vi "_Main_01.vi"() -> ()   [LabVIEW 2017]
uses:
  <vilib>/Instr/_visa.llb/VISA Configure Serial Port (Instr).vi
  <vilib>/Analysis/NI_AALBase.lvlib
panel:
  in  "Numeric":dbl min=0.0 max=11.73
  in  "OK Button":bool
  out "3 sd":dbl format="%0.2f"
  out "mean":dbl format="%0.2f"
  out "TrigTimer, s":dbl
  out "Histogram Graph":T1(graph)
  out "temp":dbl format="%#.2g"
  out "serv1":i32
  out "serv2":i32
  out "serv3":i32
  out "serv4":i32
  out "Vout, V":dbl format="%#.2g"
  out "Vin, V":dbl format="%#.3g"
  out "Temp, K":dbl
  out "Temp_sp, K":dbl
  out "Temp_gsp, K":dbl
  out "Field LOG":cluster{dbl[], dbl[]}(graph)
  out "Bytes at Port":u32
  out "RecTry":i32
  in  "Stop Button":bool
  in  "COM port":refnum<visa-resource-name>
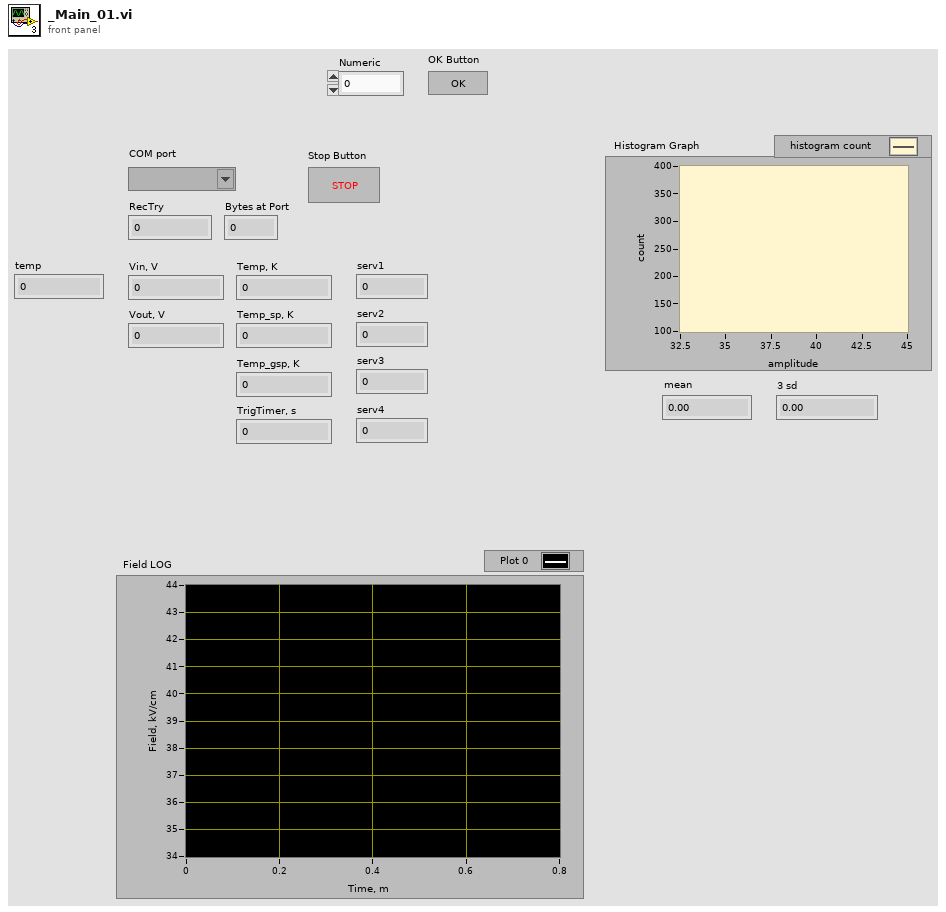
[diagram p1: front panel]
types:
  T1 = cluster{"X Values":dbl[], "Histogram: h(x)":i32[]}
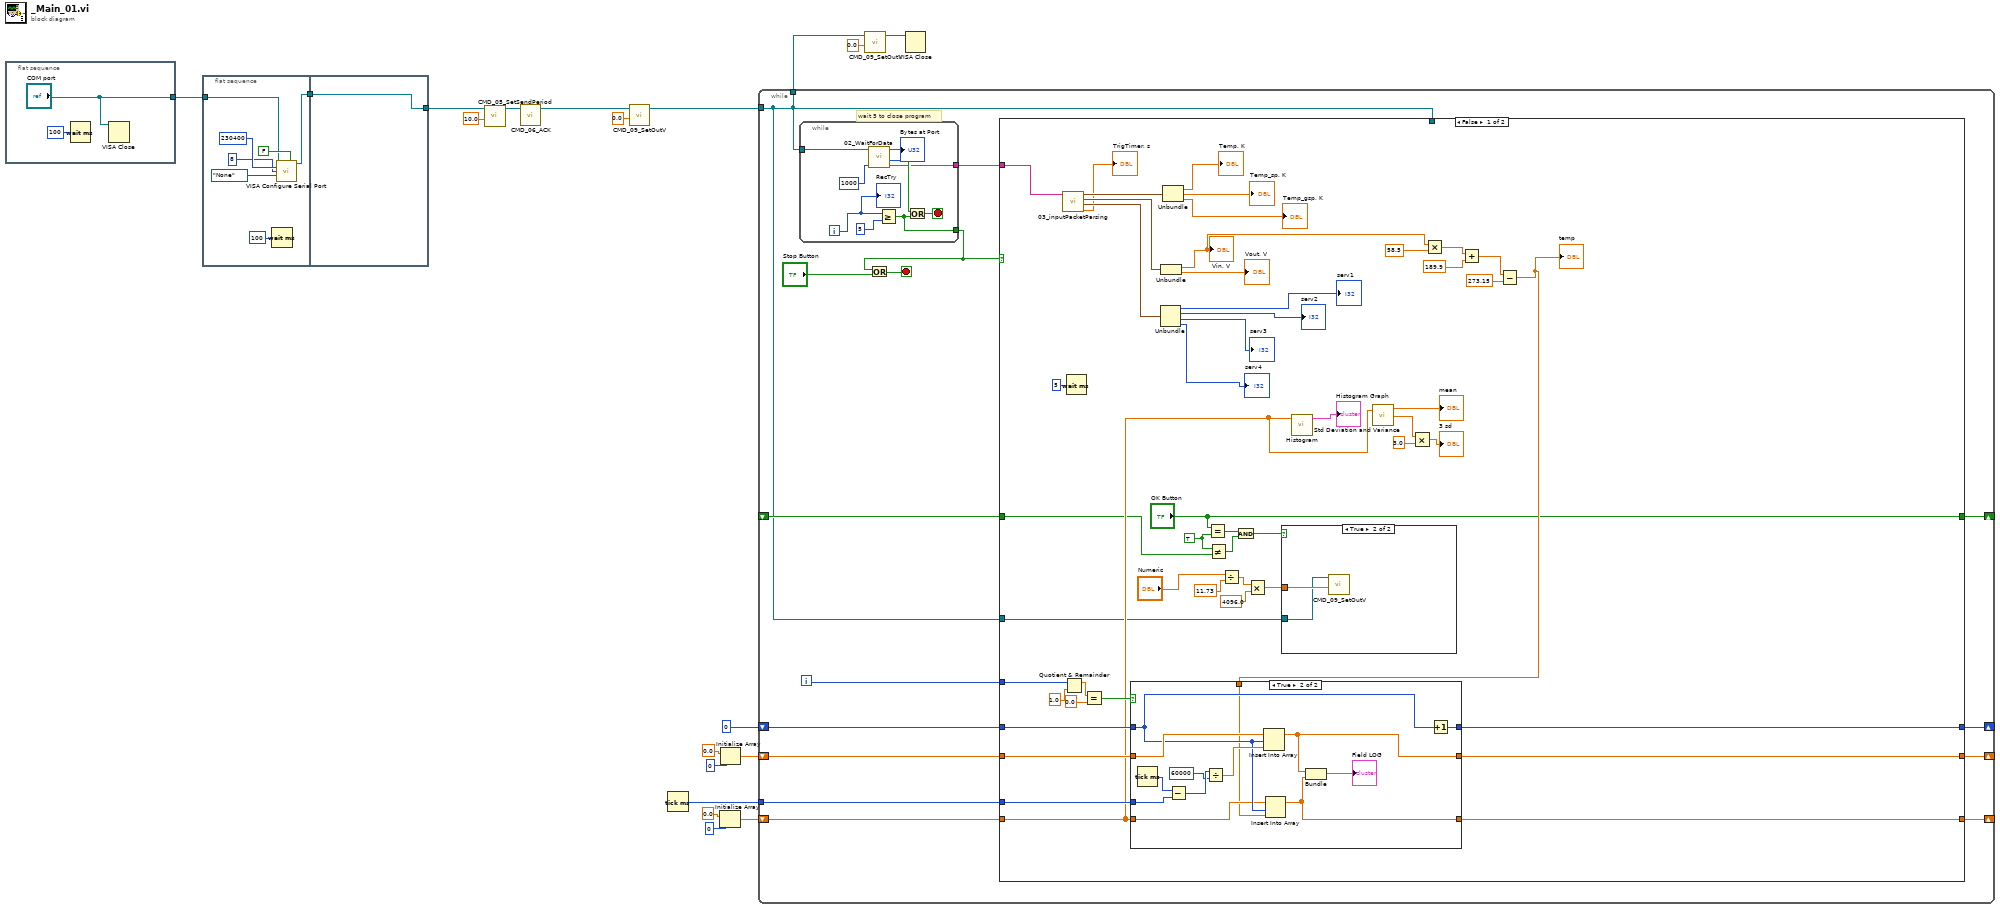
[diagram p0: block diagram]
diagram:
  n1 = flat-sequence {
    tunnel: ["COM port"] -> w19
    frame #0 {
      n2 = Wait (ms)(milliseconds to wait=u32 100) -> ()  [unwired: 1 out]
      n3 = VISA Close(VISA resource name="COM port") -> ()  [unwired: 1 in, 1 out]
    }
  }
  n4 = flat-sequence {
    tunnel: w19 -> [w24]
    tunnel: [w23] -> w16
    tunnel: [w29] -> w7
    tunnel: w16 -> [w29]
    frame #0 {
      n5 = Wait (ms)(milliseconds to wait=u32 100) -> ()  [unwired: 1 out]
      n6 = call-poly "VISA Configure Serial Port"("VISA resource name"=w24, "Enable Termination\nChar (T)"=FALSE ("Enable Termination\nChar (T)"), "baud rate (9600)"=u32 230400, "data bits (8)"=u16 8, "parity (0:none)"=enum16{"None", "Odd", "Even", "Mark", "Space"}."None") -> ("VISA resource name out"=w23:refnum<visa-resource-name>)  [unwired: 9 in, 1 out]
    }
    frame #1 {
    }
  }
  n7 = call "CMD_05_SetSendPeriod.vi"("Period, ms"=10.0, "VISA resource name"=w7) -> ("VISA resource name out"=w17:refnum<visa-resource-name>)  [unwired: 9 in]
  n8 = call "CMD_06_ACK.vi"("VISA resource name"=w17) -> ("VISA resource name out"=w1:refnum<visa-resource-name>)  [unwired: 10 in]
  n9 = call "CMD_09_SetOutV.vi"("Voltage, d"=0.0, "VISA resource name"=w1) -> ("VISA resource name out"=w2:refnum<visa-resource-name>)  [unwired: 9 in]
  n10 = Tick Count (ms)() -> (millisecond timer value=w11:u32)
  n11 = Initialize Array(0.0 ("element"), 0 ("dimension size")) -> (w8:dbl[])
  n12 = Initialize Array(0.0 ("element"), 0 ("dimension size")) -> (w12:dbl[])
  n13 = while {
    tunnel: w2 -> [w30]
    tunnel: [w30] -> w5
    shift-right: [w39] -> _
    shift-left: 0 -> [w40]
    tunnel: w11 -> [w37]
    shift-right: [w35] -> _
    shift-left: w12 -> [w38]
    shift-right: [w34] -> _
    shift-left: w8 -> [w36]
    shift-right: [w32] -> _
    shift-left: _ -> [w31]
    i -> [w41]
    stop <- w44 stop-if-true
    # "wait 5 to close program"
    n14 = while {
      tunnel: w30 -> [w117]
      tunnel: [w120] -> w43
      tunnel: [w121] -> w42
      i -> [w119]
      stop <- w123 stop-if-true
      n15 = call "02_WaitForData.vi"("WaitTimeoutMS"=u32 1000, "VISA"=w117) -> ("Buffer"=w121:string, "Bytes at Port"=→"Bytes at Port":u32, "Data Recived"=w122:bool)  [unwired: 7 in]
      n16 = Greater Or Equal?(x=w119, y=5) -> (x >= y?=w120:bool)
      n17 = Or(x=w122, y=w120) -> (x .or. y?=w123:bool)
      "RecTry" <- w119
    }
    n18 = Or(x=w43, y="Stop Button") -> (x .or. y?=w44:bool)
    n19 = case shown="False" w43 {
      tunnel: w42 -> [w84 _]
      tunnel: w41 -> [w91 _]
      tunnel: w30 -> [_ _]
      tunnel: w40 -> [w89 w116]
      tunnel: [w88 w116] -> w39
      tunnel: w38 -> [w64 w115]
      tunnel: w37 -> [w87 _]
      tunnel: w36 -> [w61 w114]
      tunnel: [w86 w115] -> w35
      tunnel: [w85 w114] -> w34
      tunnel: ["OK Button" w113] -> w32
      tunnel: w31 -> [w54 w113]
      tunnel: w30 -> [w50 _]
      frame False {
        w53 = TRUE ("x")
        n20 = call "03_inputPacketParsing.vi"("string"=w84) -> ("TrigTimer, s"=→"TrigTimer, s":dbl, "Service"=w76:cluster{i32, i32, i32, i32}, "Voltage"=w78:cluster{dbl, dbl}, "Temp"=w82:cluster{dbl, dbl, dbl})  [unwired: 7 in]
        n21 = Quotient & Remainder(x=w91, y=1.0) -> (x-y*floor(x/y)=w94:dbl)  [unwired: 1 out]
        n22 = Wait (ms)(milliseconds to wait=u32 5) -> ()  [unwired: 1 out]
        n23 = Equal?(x=w94, y=0.0) -> (x = y?=w90:bool)
        n24 = Unbundle(w76) -> (→"serv1":i32, →"serv2":i32, →"serv3":i32, →"serv4":i32)
        n25 = Unbundle(w78) -> (w71:dbl, →"Vout, V":dbl)
        "Vin, V" <- w71
        n26 = Unbundle(w82) -> (→"Temp, K":dbl, →"Temp_sp, K":dbl, →"Temp_gsp, K":dbl)
        n27 = Equal?(x="OK Button", y=w53) -> (x = y?=w56:bool)
        n28 = Not Equal?(x=w53, y=w54) -> (x != y?=w52:bool)
        n29 = Divide(x="Numeric", y=11.73) -> (x/y=w48:dbl)
        n30 = And(x=w56, y=w52) -> (x .and. y?=w51:bool)
        n31 = Multiply(x=w48, y=4096.0) -> (x*y=w46:dbl)
        n32 = case shown="True" w51 {
          tunnel: w46 -> [_ w96]
          tunnel: w50 -> [_ w95]
          frame False {
          }
          frame True {
            n33 = call "CMD_09_SetOutV.vi"("Voltage, d"=w96, "VISA resource name"=w95) -> ()  [unwired: 9 in, 1 out]
          }
        }
        n34 = call <vilib>:"Histogram.vi"("X"=w61) -> ("Histogram Graph"=→"Histogram Graph":T1)  [unwired: 7 in, 3 out]
        n35 = call <vilib>:"Std Deviation and Variance.vi"("X"=w61) -> ("mean"=→"mean":dbl, "standard deviation"=w59:dbl)  [unwired: 1 in, 1 out]
        n36 = Multiply(x=w59, y=3.0) -> (x*y=→"3 sd":dbl)
        n37 = Multiply(x=w71, y=58.5) -> (x*y=w69:dbl)
        n38 = Add(x=w69, y=189.9) -> (x+y=w67:dbl)
        n39 = Subtract(x=w67, y=273.15) -> (x-y=w65:dbl)
        "temp" <- w65
        n40 = case shown="True" w90 {
          tunnel: w89 -> [w99 w105]
          tunnel: [w99 w108] -> w88
          tunnel: w64 -> [w97 w106]
          tunnel: w87 -> [_ w111]
          tunnel: w61 -> [w98 w104]
          tunnel: [w98 w102] -> w85
          tunnel: [w97 w101] -> w86
          tunnel: w65 -> [_ w100]
          frame False {
          }
          frame True {
            n41 = Tick Count (ms)() -> (millisecond timer value=w112:u32)
            n42 = Subtract(x=w112, y=w111) -> (x-y=w110:u32)
            n43 = Divide(x=w110, y=u32 60000) -> (x/y=w107:dbl)
            n44 = Insert Into Array(array=w106, index=w105, new element=w107) -> (w101:dbl[])
            n45 = Insert Into Array(array=w104, index=w105, new element=w100) -> (w102:dbl[])
            n46 = Bundle(w101, w102) -> (→"Field LOG":cluster{dbl[], dbl[]})  [unwired: 1 in]
            n47 = Increment(x=w105) -> (x+1=w108:i32)
          }
        }
      }
      frame True {
      }
    }
  }
  n48 = call "CMD_09_SetOutV.vi"("Voltage, d"=0.0, "VISA resource name"=w5) -> ("VISA resource name out"=w6:refnum<visa-resource-name>)  [unwired: 9 in]
  n49 = VISA Close(VISA resource name=w6) -> ()  [unwired: 1 in, 1 out]
